vi "epsilonMaszynowy.vi"() -> ()   [LabVIEW 2024]
panel:
  out "Epsilon Maszynowy":dbl
  out "Waveform Graph":dbl[](graph)
  in  "Wejœcie":dbl
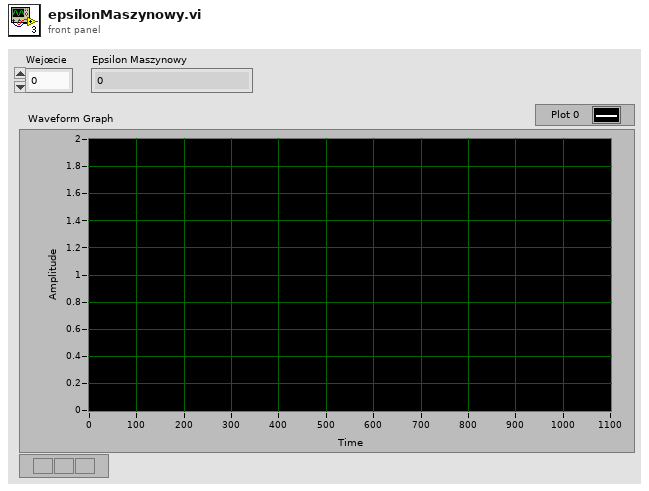
[diagram p1: front panel]
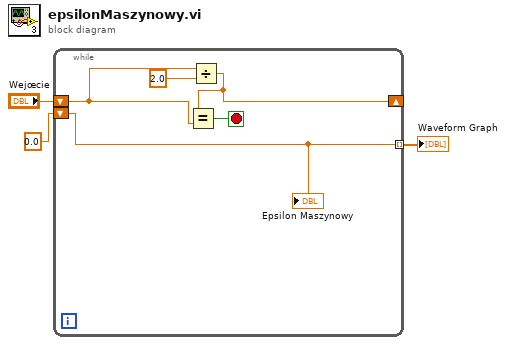
[diagram p0: block diagram]
diagram:
  n1 = while {
    shift-right: [w5] -> _
    shift-left: "Wejœcie" -> [w6]
    shift-left: 0.0 ("x") -> [w4]
    tunnel: [w4] -> w1 mode=indexing
    stop <- w8 stop-if-true
    n2 = Divide(x=w6, y=2.0) -> (x/y=w5:dbl)
    n3 = Equal?(x=w5, y=w6) -> (x = y?=w8:bool)
    "Epsilon Maszynowy" <- w4
  }
  "Waveform Graph" <- w1
